vi "Init.vi"(7 "I2C #":T1=-1, 8 "error in (no error)":errorcluster, 10 "Session In":refnum<class "Session.lvclass">) -> (0 "error out":errorcluster, 2 "2D Picture":picture, 3 "48x64 I2C OLED SSD1306 Out":refnum<class "48x64 I2C OLED SSD1306.lvclass">)   [LabVIEW 2020, in "CTI-Peripheral.lvlib" / "48x64 I2C OLED SSD1306.lvclass"]
uses:
  48x64 I2C OLED SSD1306.lvclass
  CTI/Session/Session.lvclass
  CTI/I2C Number.ctl
  CTI/I2C Address.ctl
  Data Types/OLED Size.ctl
  CTI/I2C Connection/I2C Connection.lvclass/I2C Connection.ctl
  48x64 I2C OLED SSD1306.lvclass/48x64 I2C OLED SSD1306.ctl
  CTI/I2C Connection/I2C Connection.lvclass
  CTI/CTI.lvlib
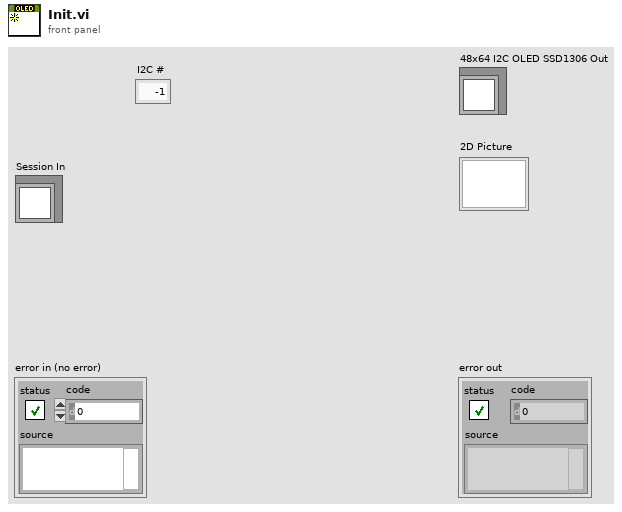
[diagram p1: front panel]
types:
  T1 = typedef "CTI.lvlib/I2C Number.ctl" = i8
  T2 = typedef "CTI-Peripheral.lvlib/48x64 I2C OLED SSD1306.lvclass/OLED Size.ctl" = cluster{"Rows":u8, "Cols":u8}
  T3 = typedef "CTI.lvlib/I2C Address.ctl" = u8
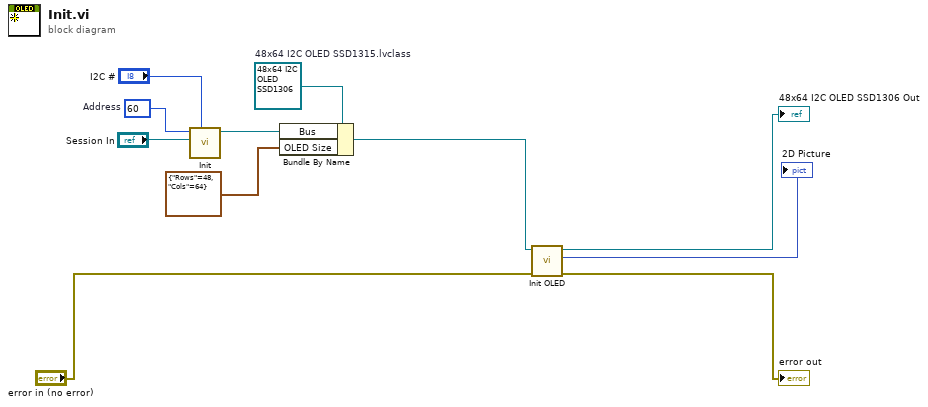
[diagram p0: block diagram]
diagram:
  w7 = refnum<class "48x64 I2C OLED SSD1306.lvclass"> refnum  # 48x64 I2C OLED SSD1315.lvclass
  w8 = T3 60  # Address
  n1 = call "Init.vi"("I2C #"="I2C #", "Session"="Session In", "Address"=w8) -> ("I2C Connection"=w11:refnum<class "I2C Connection.lvclass">)  [unwired: 7 in, 1 out]
  n2 = Bundle By Name(cluster=w7, "Bus"=w11, "OLED Size"=T2 {"Rows"=48, "Cols"=64}) -> (w5:refnum<class "48x64 I2C OLED SSD1306.lvclass">)
  n3 = call "Init OLED.vi"("error in (no error)"="error in (no error)", "48x64 I2C OLED SSD1306 in"=w5) -> ("error out"=→"error out":errorcluster, "2D Picture"=→"2D Picture":picture, "48x64 I2C OLED SSD1306 out"=→"48x64 I2C OLED SSD1306 Out":refnum<class "48x64 I2C OLED SSD1306.lvclass">)  [unwired: 7 in]
